vi "Setup subWorkers.vi"(8 "error in":errorcluster, 11 "Main View in":refnum<class "Main View.lvclass">) -> (0 "error out":errorcluster, 3 "Main View out":refnum<class "Main View.lvclass">)   [LabVIEW 2018, in "Main View.lvclass"]
doc: "<b>Note: Do not change the code in this VI!</b>\nThis VI performs a setup of all the statically-linked subWorkers that belong to the Worker that calls this VI. This VI is created automatically by the 'Create/Add Worker' tool and must be called <b>before</b> any statically linked subWorkers are called."
uses:
  Main View.lvclass
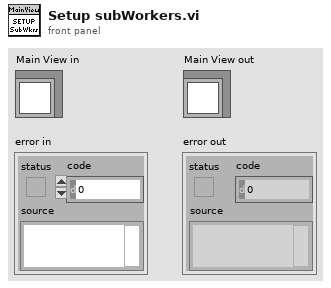
[diagram p1: front panel]
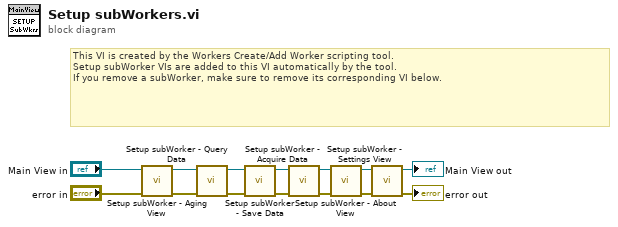
[diagram p0: block diagram]
diagram:
  # "This VI is created by the Workers Create/Add Worker scripting tool.\nSetup subWorker VIs are added to this VI automatically by the tool.\nIf you remove a subWorker, make sure to remove its corresponding VI below."
  n1 = call "Setup subWorker - Aging View.vi"("error in"="error in", "Main View in"="Main View in") -> ("error out"=w13:errorcluster, "Main View out"=w10:refnum<class "Main View.lvclass">)  [unwired: 8 in]
  n2 = call "Setup subWorker - Query Data.vi"("error in"=w13, "Main View in"=w10) -> ("error out"=w11:errorcluster, "Main View out"=w8:refnum<class "Main View.lvclass">)  [unwired: 8 in]
  n3 = call "Setup subWorker - Save Data.vi"("error in"=w11, "Main View in"=w8) -> ("error out"=w9:errorcluster, "Main View out"=w6:refnum<class "Main View.lvclass">)  [unwired: 8 in]
  n4 = call "Setup subWorker - Acquire Data.vi"("error in"=w9, "Main View in"=w6) -> ("error out"=w7:errorcluster, "Main View out"=w4:refnum<class "Main View.lvclass">)  [unwired: 8 in]
  n5 = call "Setup subWorker - About View.vi"("error in"=w7, "Main View in"=w4) -> ("error out"=w5:errorcluster, "Main View out"=w2:refnum<class "Main View.lvclass">)  [unwired: 8 in]
  n6 = call "Setup subWorker - Settings View.vi"("error in"=w5, "Main View in"=w2) -> ("error out"=→"error out":errorcluster, "Main View out"=→"Main View out":refnum<class "Main View.lvclass">)  [unwired: 8 in]
